vi "is a.vi"(8 "error in (no error)":errorcluster, 11 "PSU in":refnum<class "PSU.lvclass">) -> (0 "error out":errorcluster, 2 "is a":string, 3 "PSU out":refnum<class "PSU.lvclass">)   [LabVIEW 2026, in "Hardware.lvlib" / "PSU.lvclass"]
uses:
  PSU.lvclass
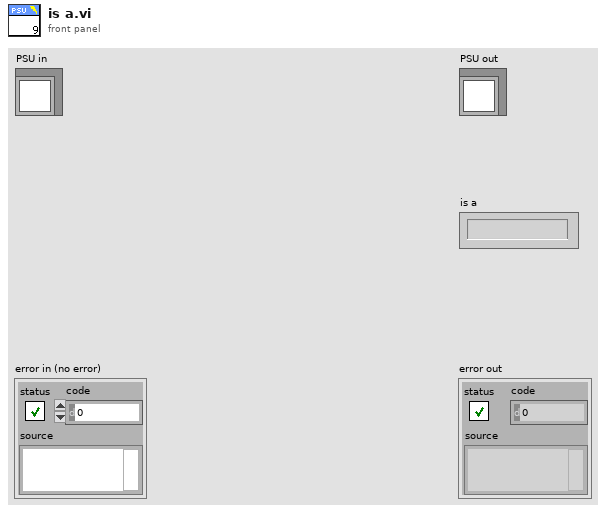
[diagram p1: front panel]
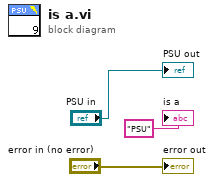
[diagram p0: block diagram]
diagram:
  "error out" <- "error in (no error)"
  "PSU out" <- "PSU in"
  "is a" <- "PSU" ("is a")
